vi "Log_create_logFile_default.vi"(11 "appdir":path) -> (0 "errout":errorcluster caption="sortie d'erreur", 3 "Fichier à flux d'octets en sortie":refnum<file>)   [LabVIEW 2020]
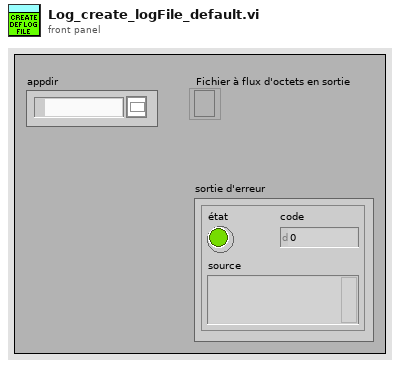
[diagram p1: front panel]
types:
  T1 = enum16{"open", "replace", "create", "open or create", "replace or create", "replace or create with confirmation"}
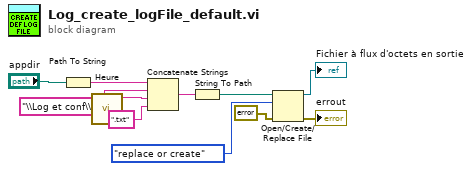
[diagram p0: block diagram]
diagram:
  n1 = Path To String(path="appdir") -> (string=w10:string)
  n2 = call "Heure.vi"() -> ("chaîne concaténée"=w3:string)  [unwired: 11 in]
  n3 = Concatenate Strings(w10, "\\Log et conf\\", w3, ".txt" ("chaîne")) -> (w5:string)
  n4 = String To Path(string=w5) -> (path=w6:path)
  n5 = Open/Create/Replace File(file path (use dialog)=w6, error in=errorcluster {"status"=FALSE, "code"=0, "source"=""} ("entrée d'erreur"), operation (0:open)=T1."replace or create" ("opération (0 : open)")) -> (refnum out=→"Fichier à flux d'octets en sortie":refnum<file>, error out=→"errout":errorcluster)  [unwired: 3 in, 1 out]
